vi "FTW-XML-Element-Add.vi"(0 "Document":refnum<k20>, 5 "XML Element to Add":string, 11 "error in":errorcluster) -> (4 "Document out":refnum<k20>, 6 "New Element":refnum<k20>, 15 "error out":errorcluster)   [LabVIEW 2015]
uses:
  <resource>/objmgr/DOMUserDefRef.rc
panel:
  # "Inputs"
  # "Outputs"
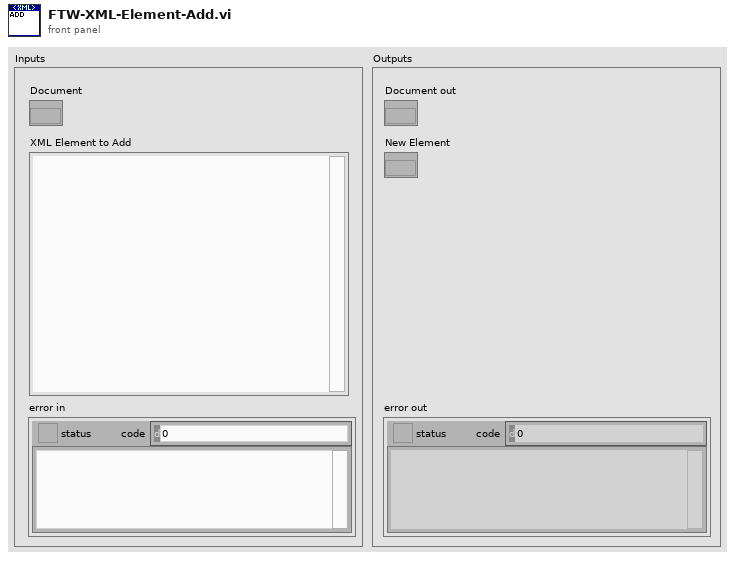
[diagram p1: front panel]
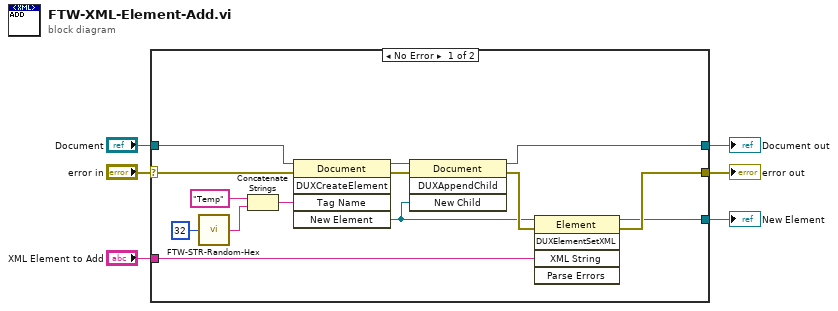
[diagram p0: block diagram]
diagram:
  n1 = case shown="No Error" "error in" {
    selector: "error in" -> [w20 w22]
    tunnel: [w9 w22] -> w6
    tunnel: "Document" -> [w18 w21]
    tunnel: [w16 w21] -> w3
    tunnel: "XML Element to Add" -> [w17 _]
    tunnel: [w7 _] -> w1
    frame No Error {
      n2 = call "FTW-STR-Random-Hex.vi"("String Length"=32) -> ("Random Hex String"=w14:string)  [unwired: 3 in]
      n3 = Concatenate Strings("Temp" ("string"), w14) -> (w12:string)
      n4 = invoke class="Document" method="DUXCreateElement"(reference=w18, error in=w20, "Tag Name"=w12) -> (reference out=w19:refnum<k20>, error out=w11:errorcluster, "New Element"=w8:refnum<k20>)  [unwired: 2 in, 2 out]
      n5 = invoke class="Document" method="DUXAppendChild"(reference=w19, error in=w11, "New Child"=w8) -> (reference out=w16:refnum<k20>, error out=w10:errorcluster)  [unwired: 1 in, 2 out]
      n6 = invoke class="Element" method="DUXElementSetXML"(reference=w8, error in=w10, "XML String"=w17) -> (reference out=w7:refnum<k20>, error out=w9:errorcluster)  [unwired: 2 in, 3 out]
    }
    frame Error {
    }
  }
  "error out" <- w6
  "Document out" <- w3
  "New Element" <- w1
